vi "Configure Minor Frame.vi"(8 "Error in (no error)":errorcluster, 9 "Transfer IDs":u16[](array[numeric]), 10 "Minor Frame ID in":u8=1, 11 "Module Handle in":u32) -> (0 "Error out":errorcluster, 2 "Minor Frame ID out":u8=1, 3 "Module Handle out":u32)   [LabVIEW 2020, in "AIM MIL-STD-1553 Hardware API.lvlib"]
uses:
  AIM MIL-STD-1553 Hardware API.lvlib
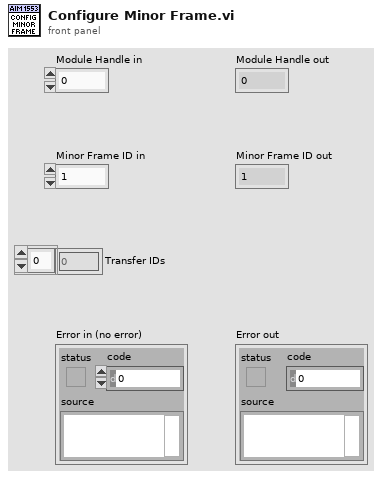
[diagram p1: front panel]
types:
  T1 = enum16{"n/a", "Normal transfer", "Skip (no op)", "Wait for time delay", "Strobe trigger"}
  T2 = cluster{"Instruction":enum16{"n/a", "Normal transfer", "Skip (no op)", "Wait for time delay", "Strobe trigger"}, "Numeric":u16}
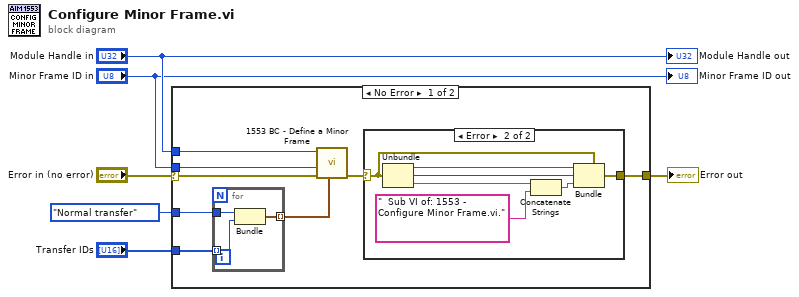
[diagram p0: block diagram]
diagram:
  n1 = case shown="No Error" "Error in (no error)" {
    tunnel: "Minor Frame ID in" -> [w8 _]
    selector: "Error in (no error)" -> [w14 w26]
    tunnel: [w10 w26] -> w6
    tunnel: "Transfer IDs" -> [w13 _]
    tunnel: T1."Normal transfer" ("Instruction") -> [w12 _]
    tunnel: "Module Handle in" -> [w9 _]
    frame No Error {
      n2 = for {
        tunnel: w13 -> [w16] mode=indexing
        tunnel: w12 -> [w17]
        tunnel: [w15] -> w11 mode=indexing
        n3 = Bundle("Instruction"=w17, "Numeric"=w16) -> (w15:T2)  [unwired: 1 in]
      }
      n4 = call <instrlib>:"1553 BC - Define a Minor Frame.vi"("Transfer List"=w11, "Error In (none)"=w14, "Minor Frame ID (1)"=w8, "Module Handle"=w9) -> ("Error Out"=w7:errorcluster)  [unwired: 6 in, 1 out]
      n5 = case shown="Error" w7 {
        selector: w7 -> [w18 w25]
        tunnel: [w18 w22] -> w10
        frame No Error {
        }
        frame Error {
          n6 = Unbundle(w25) -> ("status"=w23:bool, "code"=w24:i32, "source"=w21:string)
          n7 = Concatenate Strings(w21, "  Sub VI of: 1553 - Configure Minor Frame.vi.") -> (w20:string)
          n8 = Bundle(cluster=w25, "status"=w23, "code"=w24, "source"=w20) -> (w22:errorcluster)
        }
      }
    }
    frame Error {
    }
  }
  "Error out" <- w6
  "Module Handle out" <- "Module Handle in"
  "Minor Frame ID out" <- "Minor Frame ID in"
